vi "LeCroy Wave Series Edge Triggered Acquisition.vi"() -> ()   [LabVIEW 2013]
doc: "This example shows how to configure the oscilloscope to perform an edge-triggered waveform acquisition."
uses:
  <instrlib>/LeCroy Wave Series/LeCroy Wave Series.lvlib
  <instrlib>/LeCroy Wave Series/Public/Configure/Configure Edge Trigger.vi
  <instrlib>/LeCroy Wave Series/Public/Data/Read Single Waveform.vi
panel:
  in  "Source (1: Channel 1)":u16(ring) items=["Channel 1", "Channel 2", "Channel 3", "Channel 4", "Memory 1", "Memory 2", "Memory 3", "Memory 4", "Function 1", "Function 2", "Function 3", "Function 4", "Function 5", "Function 6", "Function 7", "Function 8"]
  in  "Vertical Coupling (0: A1M)":u16(ring) items=["A1M", "D1M", "D50", "Ground"]
  in  "Probe Attenuation (-1)":dbl=-1.0
  in  "Vertical Range (1.0 V)":dbl=10.0
  in  "Trigger Level (0.0 V)":dbl
  in  "Timebase (0.0005 s)":dbl=0.0005
  out "Waveform Data":waveform(dbl)(graph)
  in  "Source (0: Channel 1)":u16(ring) items=["Channel 1", "Channel 2", "Channel 3", "Channel 4"]
  in  "VISA resource name":refnum<visa-resource-name>
  # "(c) 2005 - 2012 NATIONAL INSTRUMENTS.  ALL RIGHTS RESERVED."
  # "Note:\nThis VI will time out without acquiring any data if the input signal on channel 1 does not cross 0 V trigger level with positive slope.\nFor more details on triggering pleas see the Edge Triggered Acquisition Example VI."
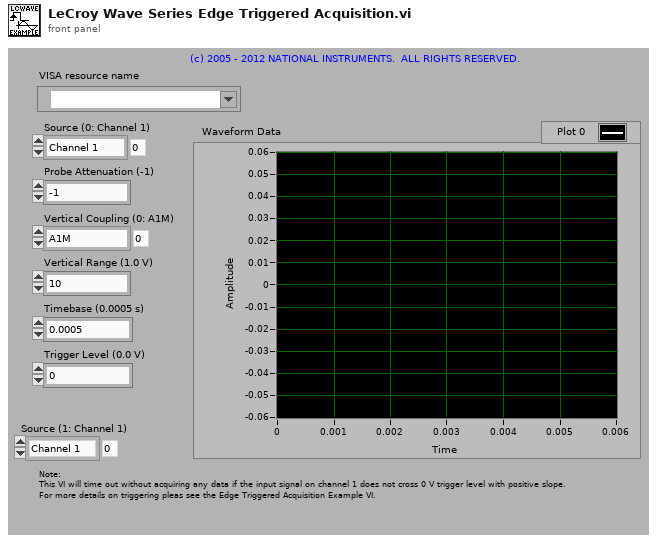
[diagram p1: front panel]
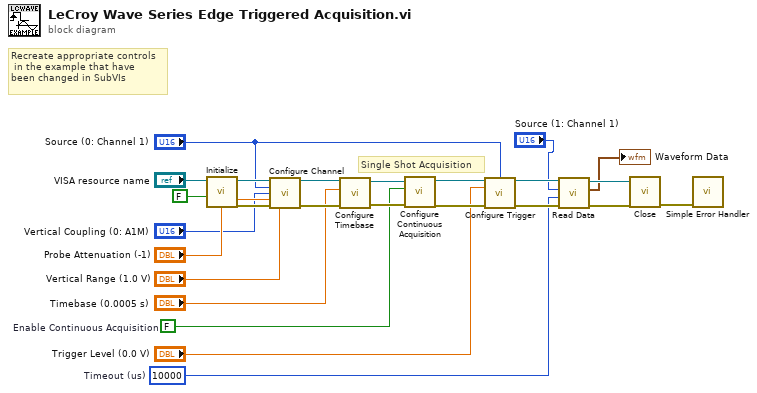
[diagram p0: block diagram]
diagram:
  w3 = u32 10000  # Timeout (us)
  w8 = FALSE  # Enable Continuous Acquisition
  # "Recreate appropriate controls\n in the example that have \nbeen changed in SubVIs"
  # "Single Shot Acquisition"
  n1 = call <instrlib>:"Initialize.vi"("Reset? (T: Yes)"=FALSE, "VISA resource name"="VISA resource name") -> ("error out"=w19:errorcluster, "VISA resource name out"=w20:refnum<visa-resource-name>)  [unwired: 8 in]
  n2 = call <instrlib>:"Configure Channel.vi"("VISA resource name"=w20, "Channel (0: Channel 1)"="Source (0: Channel 1)", "Vertical Coupling (0: A1M)"="Vertical Coupling (0: A1M)", "Enable Channel (T:On)"="Probe Attenuation (-1)", "error in (no error)"=w19, "Bandwidth (0: Full)"="Vertical Range (1.0 V)") -> ("VISA resource name out"=w23:refnum<visa-resource-name>, "error out"=w24:errorcluster)  [unwired: 8 in]
  n3 = call <instrlib>:"Configure Timebase.vi"("error in (no error)"=w24, "Timebase (0.0005 s)"="Timebase (0.0005 s)", "VISA resource name"=w23) -> ("error out"=w10:errorcluster, "VISA resource name out"=w13:refnum<visa-resource-name>)  [unwired: 7 in]
  n4 = call <instrlib>:"Configure Continuous Acquisition.vi"("error in (no error)"=w10, "Continuous Acquisition Mode (T: On)"=w8, "VISA resource name"=w13) -> ("error out"=w11:errorcluster, "VISA resource name out"=w12:refnum<visa-resource-name>)  [unwired: 7 in]
  n5 = call-poly <instrlib>:"Configure Trigger.vi"("VISA resource name"=w12, 2:"Source (0: Channel 1)", "Trigger Source (0: Channel 1)"="Trigger Level (0.0 V)", "error in (no error)"=w11) -> ("VISA resource name out"=w15:refnum<visa-resource-name>, "error out"=w14:errorcluster)  [unwired: 10 in]
  n6 = call-poly <instrlib>:"Read Data.vi"("error in (no error)"=w14, "Timeout (10000 ms)"=w3, "Source (0: Channel 1)"="Source (1: Channel 1)", "VISA resource name"=w15) -> ("error out"=w17:errorcluster, "Waveform Data"=→"Waveform Data":waveform(dbl), "VISA resource name out"=w18:refnum<visa-resource-name>)  [unwired: 5 in]
  n7 = call <instrlib>:"Close.vi"("error in (no error)"=w17, "VISA resource name"=w18) -> ("error out"=w25:errorcluster)  [unwired: 9 in]
  n8 = call <vilib>:"Simple Error Handler.vi"("error in (no error)"=w25) -> ()  [unwired: 4 in, 5 out]
